vi "Create Channel.vi"(8 "error in":errorcluster, 11 "Node In":refnum<k20>) -> (0 "error out":errorcluster, 2 "Channel out":refnum<class "Channel.lvclass">, 3 "Node out":refnum<k20>)   [LabVIEW 2024, in "Parser.lvlib" / "Channel.lvclass"]
uses:
  Channel.lvclass
  Channel.lvclass/Channel.ctl
  Item/Item.lvclass/Item.ctl
  Item/Write Properties.vi
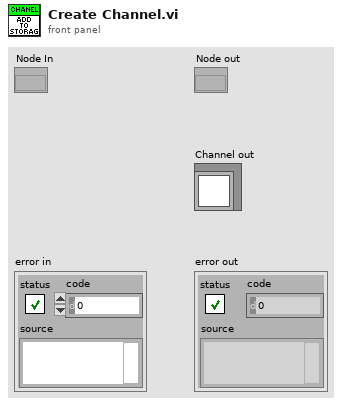
[diagram p1: front panel]
types:
  T1 = cluster{"DefaultValue":dbl, "Errors":cluster{"Key":string, "IsError":bool, "Code":u32, "Message":string}[], "Description":string}
  T2 = cluster{"Name":string, "Type":enum16{"Input", "Output"}, "TypeGUID":string, "Identifier":string, "RowDim":i32, "ColDim":i32, "Units":string, "Scalable":bool, "Faultable":bool}
  T3 = cluster{"Key":string, "IsError":bool, "Code":u32, "Message":string}[]
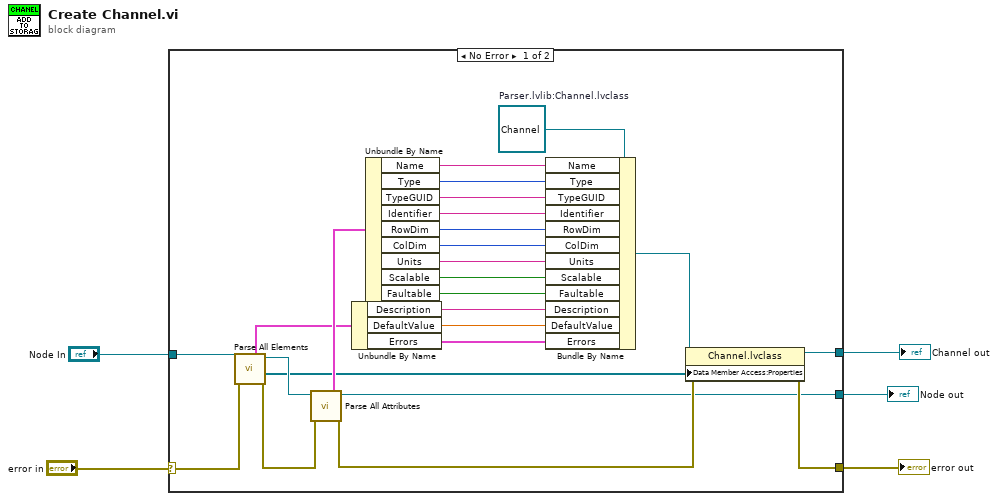
[diagram p0: block diagram]
diagram:
  n1 = case shown="No Error" "error in" {
    selector: "error in" -> [w30 w32]
    tunnel: [w27 w32] -> w4
    tunnel: "Node In" -> [w26 w31]
    tunnel: [w10 _] -> w2
    tunnel: [w7 w31] -> w1
    frame No Error {
      w24 = refnum<class "Channel.lvclass"> refnum  # Parser.lvlib:Channel.lvclass
      n2 = call "Parse All Elements.vi"("error in"=w30, "Node in"=w26) -> ("error out"=w29:errorcluster, "Properties out"=w6:refnum<class "Property.lvclass">[], "Channel Data"=w8:T1, "Node out"=w25:refnum<k20>)  [unwired: 6 in]
      n3 = call "Parse All Attributes.vi"("error in"=w29, "Node in"=w25) -> ("error out"=w28:errorcluster, "Channel Data"=w9:T2, "Node out"=w7:refnum<k20>)  [unwired: 7 in]
      n4 = Unbundle By Name(w8) -> ("Description"=w14:string, "DefaultValue"=w13:dbl, "Errors"=w12:T3)
      n5 = Unbundle By Name(w9) -> ("Name"=w23:string, "Type"=w22:enum16{"Input", "Output"}, "TypeGUID"=w21:string, "Identifier"=w20:string, "RowDim"=w19:i32, "ColDim"=w18:i32, "Units"=w17:string, "Scalable"=w16:bool, "Faultable"=w15:bool)
      n6 = Bundle By Name(cluster=w24, "Name"=w23, "Type"=w22, "TypeGUID"=w21, "Identifier"=w20, "RowDim"=w19, "ColDim"=w18, "Units"=w17, "Scalable"=w16, "Faultable"=w15, "Description"=w14, "DefaultValue"=w13, "Errors"=w12) -> (w11:refnum<class "Channel.lvclass">)
      n7 = property class="Channel.lvclass"(reference=w11, error in=w28, "Data Member Access:Properties"=w6) -> (reference out=w10:refnum<class "Channel.lvclass">, error out=w27:errorcluster)
    }
    frame Error {
    }
  }
  "error out" <- w4
  "Channel out" <- w2
  "Node out" <- w1
